vi "Update Start New File Channel.vi"(6 "New File Event":refnum<user-event>, 8 "error in (no error)":errorcluster, 10 "Command Values in":dbl[](array[numeric]), 11 "Log Info in":T1 {"Node ID" format="%.0x"; "TDMS Error Code"."Data Ref" format="%.0x"; "Missed Samples"."Data Ref" format="%.0x"; "File Status"."Data Ref" format="%.0x"; "Start New File"."Data Ref" format="%.0x"; "Logging Enabled"."Data Ref" format="%.0x"; "Stop Trigger"."Node Data Ref" format="%.0x"; "Stop Trigger"."Node ID" format="%.0x"; "Start Trigger"."Node Data Ref" format="%.0x"; "Start Trigger"."Node ID" format="%.0x"}) -> (0 "error out":errorcluster, 2 "Command Values out":dbl[](array[numeric]), 3 "Log Info out":T1 {"Node ID" format="%.0x"; "TDMS Error Code"."Data Ref" format="%.0x"; "Missed Samples"."Data Ref" format="%.0x"; "File Status"."Data Ref" format="%.0x"; "Start New File"."Data Ref" format="%.0x"; "Logging Enabled"."Data Ref" format="%.0x"; "Stop Trigger"."Node Data Ref" format="%.0x"; "Stop Trigger"."Node ID" format="%.0x"; "Start Trigger"."Node Data Ref" format="%.0x"; "Start Trigger"."Node ID" format="%.0x"})   [LabVIEW 2015, in "Waveform Data Logger Engine.lvlib"]
uses:
  Waveform Data Logger Engine.lvlib
  Types/Inline Waveform Log Info.ctl
  Classes/Log File Specifications/Waveform TDMS Log File Specification/Waveform TDMS Log File Specification.lvclass
  Classes/Triggers/Trigger/Trigger.lvclass
  <vilib>/NI Veristand/Custom Device API/Custom Device Item Ref.ctl
  Types/Inline Log Waveform.ctl
  Types/Trigger Settings.ctl
  Types/Log Status.ctl
  Types/Channel.ctl
  <vilib>/NI Veristand/Custom Device API/Data Reference.ctl
  Types/New File Event Data.ctl
  <vilib>/NI Veristand/Custom Device API/Global Data Refs.vi
  <vilib>/NI Veristand/Custom Device API/Custom Device API.lvlib
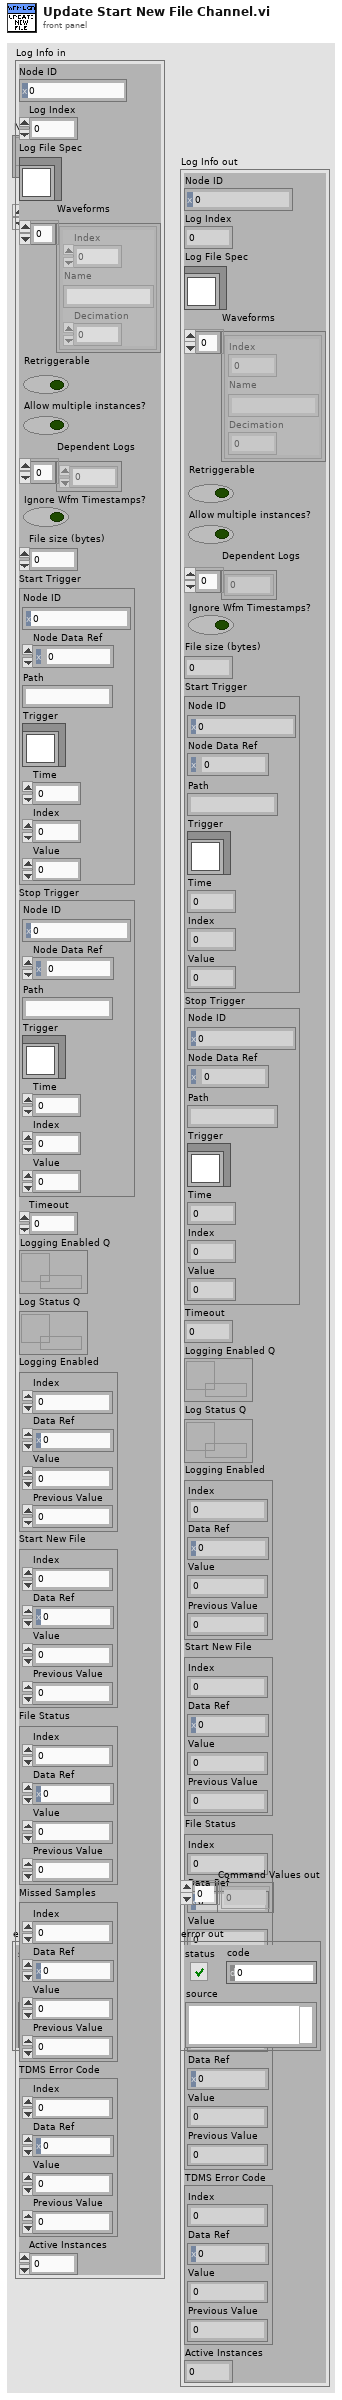
[diagram p1: front panel]
types:
  T1 = typedef "Waveform Data Logger Engine.lvlib/Inline Waveform Log Info.ctl" = cluster{"Node ID":T2, "Log Index":i32, "Log File Spec":refnum<class "Waveform TDMS Log File Specification.lvclass">, "Waveforms":T3[], "Retriggerable":bool, "Allow multiple instances?":bool, "Dependent Logs":i32[], "Ignore Wfm Timestamps?":bool, "File size (bytes)":i64, "Start Trigger":T4, "Stop Trigger":T4, "Timeout":dbl, "Logging Enabled Q":refnum<queue>, "Log Status Q":refnum<queue>, "Logging Enabled":T5, "Start New File":T5, "File Status":T5, "Missed Samples":T5, "TDMS Error Code":T5, "Active Instances":i32}
  T2 = typedef "Custom Device API.lvlib/Custom Device Item Ref.ctl" = u64
  T3 = typedef "Waveform Data Logger Engine.lvlib/Inline Log Waveform.ctl" = cluster{"Index":i32, "Name":string, "Decimation":u32}
  T4 = typedef "Waveform Data Logger Engine.lvlib/Trigger Settings.ctl" = cluster{"Node ID":T2, "Node Data Ref":i32, "Path":string, "Trigger":refnum<class "Trigger.lvclass">, "Time":dbl, "Index":i32, "Value":dbl}
  T5 = typedef "Waveform Data Logger Engine.lvlib/Channel.ctl" = cluster{"Index":i32, "Data Ref":T6, "Value":dbl, "Previous Value":dbl}
  T6 = typedef "Custom Device API.lvlib/Data Reference.ctl" = i32
  T7 = typedef "Waveform Data Logger Engine.lvlib/New File Event Data.ctl" = cluster{"Log Index":i32}
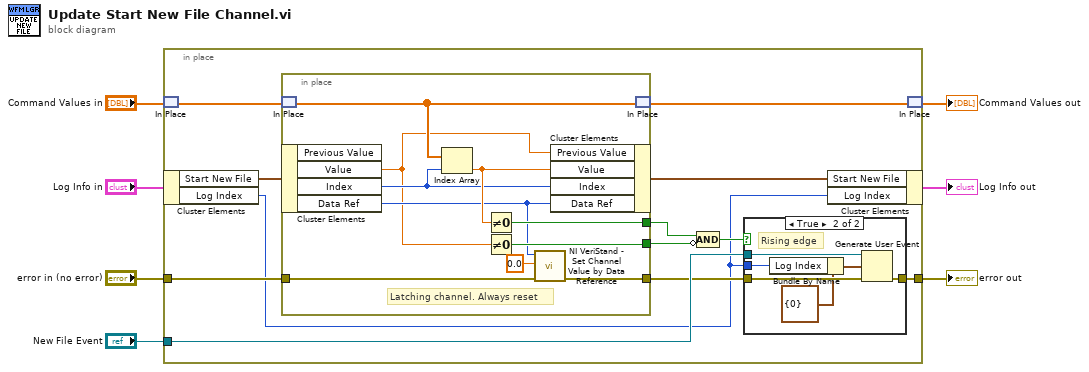
[diagram p0: block diagram]
diagram:
  n1 = in-place {
    in-place-border: [w11] -> w4
    in-place-border: "New File Event" -> [w16]
    in-place-border: "error in (no error)" -> [w9]
    n2 = in-place-match #1("Command Values in") -> (w10:dbl[])
    n3 = in-place-cluster #2("Log Info in") -> ("Start New File"=w19:T5, "Log Index"=w8:i32)
    n4 = in-place {
      in-place-border: [w33] -> w15
      in-place-border: [w32] -> w14
      in-place-border: w9 -> [w29]
      in-place-border: [w28] -> w12
      # "Latching channel. Always reset"
      n5 = in-place-match #3(w10) -> (w36:dbl[])
      n6 = in-place-cluster #4(w19) -> ("Value"=w27:dbl, "Index"=w34:i32, "Data Ref"=w30:T6)  [unwired: 1 out]
      n7 = Index Array(array=w36, index=w34) -> (element=w35:dbl)
      n8 = Not Equal To 0?(x=w35) -> (x != 0?=w33:bool)
      n9 = Not Equal To 0?(x=w27) -> (x != 0?=w32:bool)
      n10 = call <vilib>:"NI VeriStand - Set Channel Value by Data Reference.vi"("error in (no error)"=w29, "Value"=0.0, "Data Reference in"=w30) -> ("error out"=w28:errorcluster)  [unwired: 8 in]
      n11 = in-place-cluster #4("Previous Value"=w27, "Value"=w35, "Index"=w34, "Data Ref"=w30) -> (w18:T5)
      n12 = in-place-match #3(w36) -> (w17:dbl[])
    }
    n13 = Compound Arithmetic op=AND(w15, invert w14) -> (w13:bool)
    n14 = case shown="True" w13 {
      tunnel: w12 -> [w20 w26]
      tunnel: w16 -> [_ w25]
      tunnel: [w20 w24] -> w11
      tunnel: w8 -> [_ w21]
      frame False {
      }
      frame True {
        # "Rising edge"
        n15 = Bundle By Name(cluster=T7 {"Log Index"=0} ("event data"), "Log Index"=w21) -> (w23:T7)
        n16 = Generate User Event(user event=w25, event data cluster=w23, error in=w26) -> (error out=w24:errorcluster)  [unwired: 1 in, 1 out]
      }
    }
    n17 = in-place-cluster #2("Start New File"=w18, "Log Index"=w8) -> (→"Log Info out":T1)
    n18 = in-place-match #1(w17) -> (→"Command Values out":dbl[])
  }
  "error out" <- w4
